vi "KPRO_2016_DPT2.vi"() -> ()   [LabVIEW 2016]
uses:
  Kpro Globals.vi
  <vilib>/Utility/file.llb/Write To Spreadsheet File (DBL).vi
panel:
  in  "Record DTW":bool
  out "Depth to Water":dbl=-30.877198474121087 format="%.2f"
  in  "In-Line Pressure Offset":dbl format="%.2f"
  in  "Zero In-Line Pressure\n(F = leave as is)":bool=TRUE
  in  "In-Line Pressure Slope":dbl=42.0 format="%.2f"
  out "In-Line Pressure":dbl=69.7228 format="%.2f"
  out "Drive Rate":dbl=16.666666666666664 format="%.2f"
  out "Real Time - Depth vs. Drive":cluster{dbl[], dbl[]}(graph)={[0.02036245163917736, 0.125, 0.16666666666666674, 0.16666666666666663, 0.16666666666666663, 0.16666666666666663], [-100.1, -100.2, -100.3, -100.4, -100.5, -100.6]}
  out "Current Depth (m)":sgl=-30.661383 format="%.2f"
  out "Zeroed \nPressure (m)":dbl=22.78027421497274 format="%.2f"
  out "Ik":dbl=0.003788962123473114 format="%.2f"
  in  "Hole_name_file":path=path "C:/e"
  in  "Output File KPRO Test":path=path "C:/e_KPRO.txt"
  in  "Output File Slug Test":path=path "C:/e_SLUG.txt"
  in  "Output File YSI Test":path=path "C:/e_YSI.txt"
  in  "Output File IK for GMS":path=path "C:/e_IKMGS.txt"
  in  "enable_IKMGS_file":bool
  in  "enable_slug_file":bool
  in  "enable_kpro_file":bool=TRUE
  out "Ik":dbl=0.003788962123473114 format="%.2f"
  out "Zeroed Pressure":dbl=74.74207969932556 format="%.2f"
  out "Current Depth":sgl=-100.6 format="%.2f"
  out "Flow":dbl=0.21081600494384767 format="%.2f"
  out "Real Time - Depth vs. lk":cluster{dbl[], dbl[]}(graph)={[0.003788962123473114, 0.0037174584307500765, 0.0037174584307500765, 0.0037174584307500765, 0.0037174584307500765, 0.003788962123473114], [-100.1, -100.2, -100.3, -100.4, -100.5, -100.6]}
  out "Hole_Name_Path":path=path "C:/e"
  in  "data_directory":string="C:\\KPRO_DATA\\SITE_NAME\\"
  out "Real Time - Depth vs. lk":cluster{dbl[], dbl[]}(graph)={[0.003788962123473114, 0.0037174584307500765, 0.0037174584307500765, 0.0037174584307500765, 0.0037174584307500765, 0.003788962123473114], [-100.1, -100.2, -100.3, -100.4, -100.5, -100.6]}
  in  "Reservoir Pressure":dbl=-0.004827000045779073 format="%.2f"
  in  "Simulate AD6B":bool
  in  "Atmospheric Pressure":dbl=32.22022530555725 format="%.2f"
  out "numrows":dbl format="%.2f"
  in  "Start\nYSI Capture":bool
  in  "Capture Head \nPressure":bool
  in  "Depth mode":bool caption="Use \nIncrement"
  out "Real Time - Depth vs. Drive":cluster{dbl[], dbl[]}(graph)={[0.02036245163917736, 0.125, 0.16666666666666674, 0.16666666666666663, 0.16666666666666663, 0.16666666666666663], [-100.1, -100.2, -100.3, -100.4, -100.5, -100.6]}
  out "Cumulative - Depth vs. Drive":cluster{dbl[], dbl[]}(graph)
  in  "Feet of Stainless":i32=40
  out "Slug Test\nIndicator":bool
  out "KPRO Test\nIndicator":bool
  in  "Increment\nButton":bool
  in  "Start\nST":bool
  in  "Zero\nPressure":bool
  out "Zeroed \nPressure":dbl=74.74207969932556 format="%.2f"
  in  "Finish Tests":bool
  out "Current Depth":sgl=-100.6 format="%.2f"
  in  "Start\nKPRO":bool
  out "Total Volume":dbl format="%.2f"
  in  "Clear \nTotal\nVolume":bool
  in  "Client ID - Not Used":string
  out "Flow":dbl=0.21081600494384767 format="%.2f"
  out "Cumulative - Depth vs. Ik":cluster{dbl[], dbl[]}(graph)
  # "Use new slope/offset"
  # "KPRO  DATALOGGER"
  # "STONE  ENVIRONMENTAL  2010"
  # "ON"
  # "OFF"
  # "String Pot"
  # "Revision History\n\nAdded metric depth and pressure - VLD - 12-20-07\nAdded Static Ik button and drive rate- VLD 1-28-10"
  # "Use Incr"
  # "ON"
  # "OFF"
  # "ON"
  # "OFF"
  # "ON"
  # "OFF"
  # "ON"
  # "OFF"
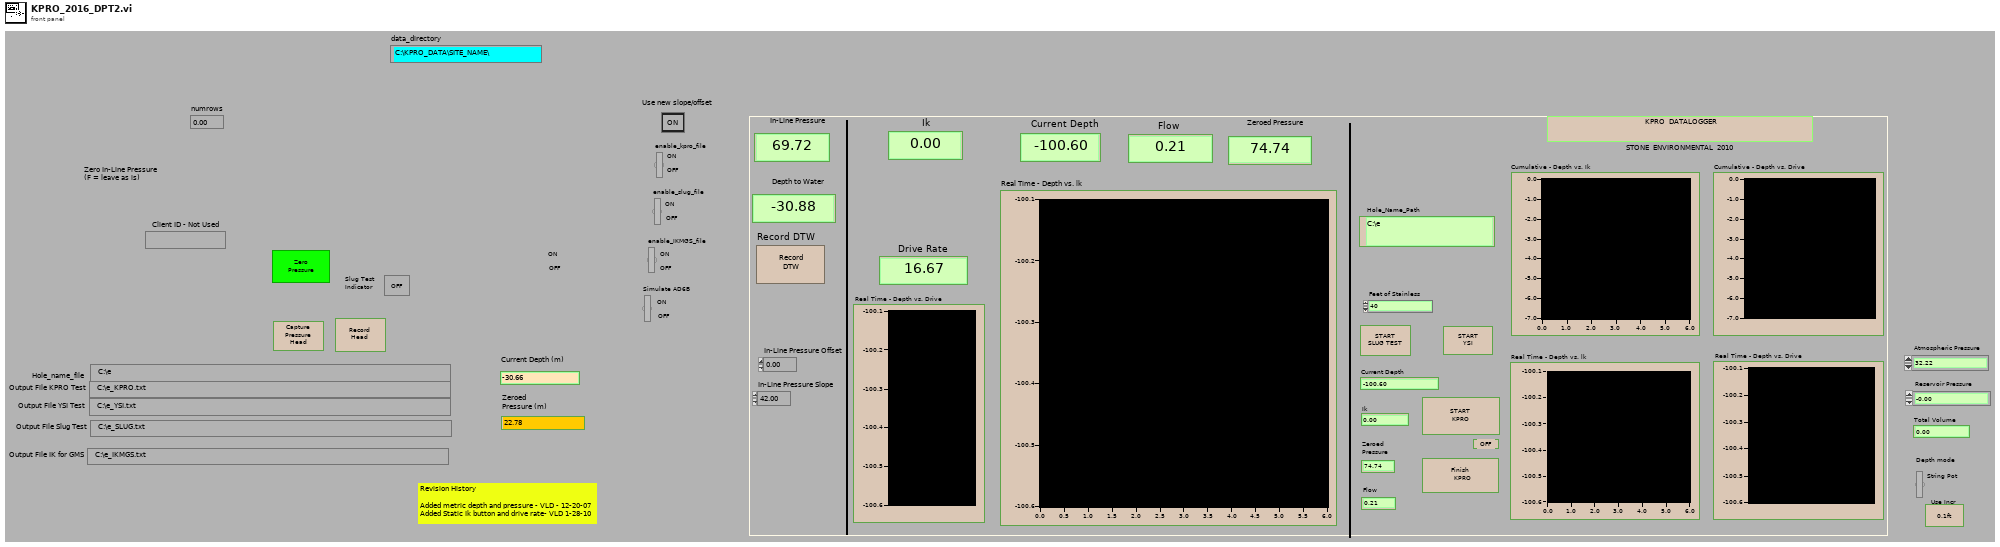
[diagram p1: front panel]
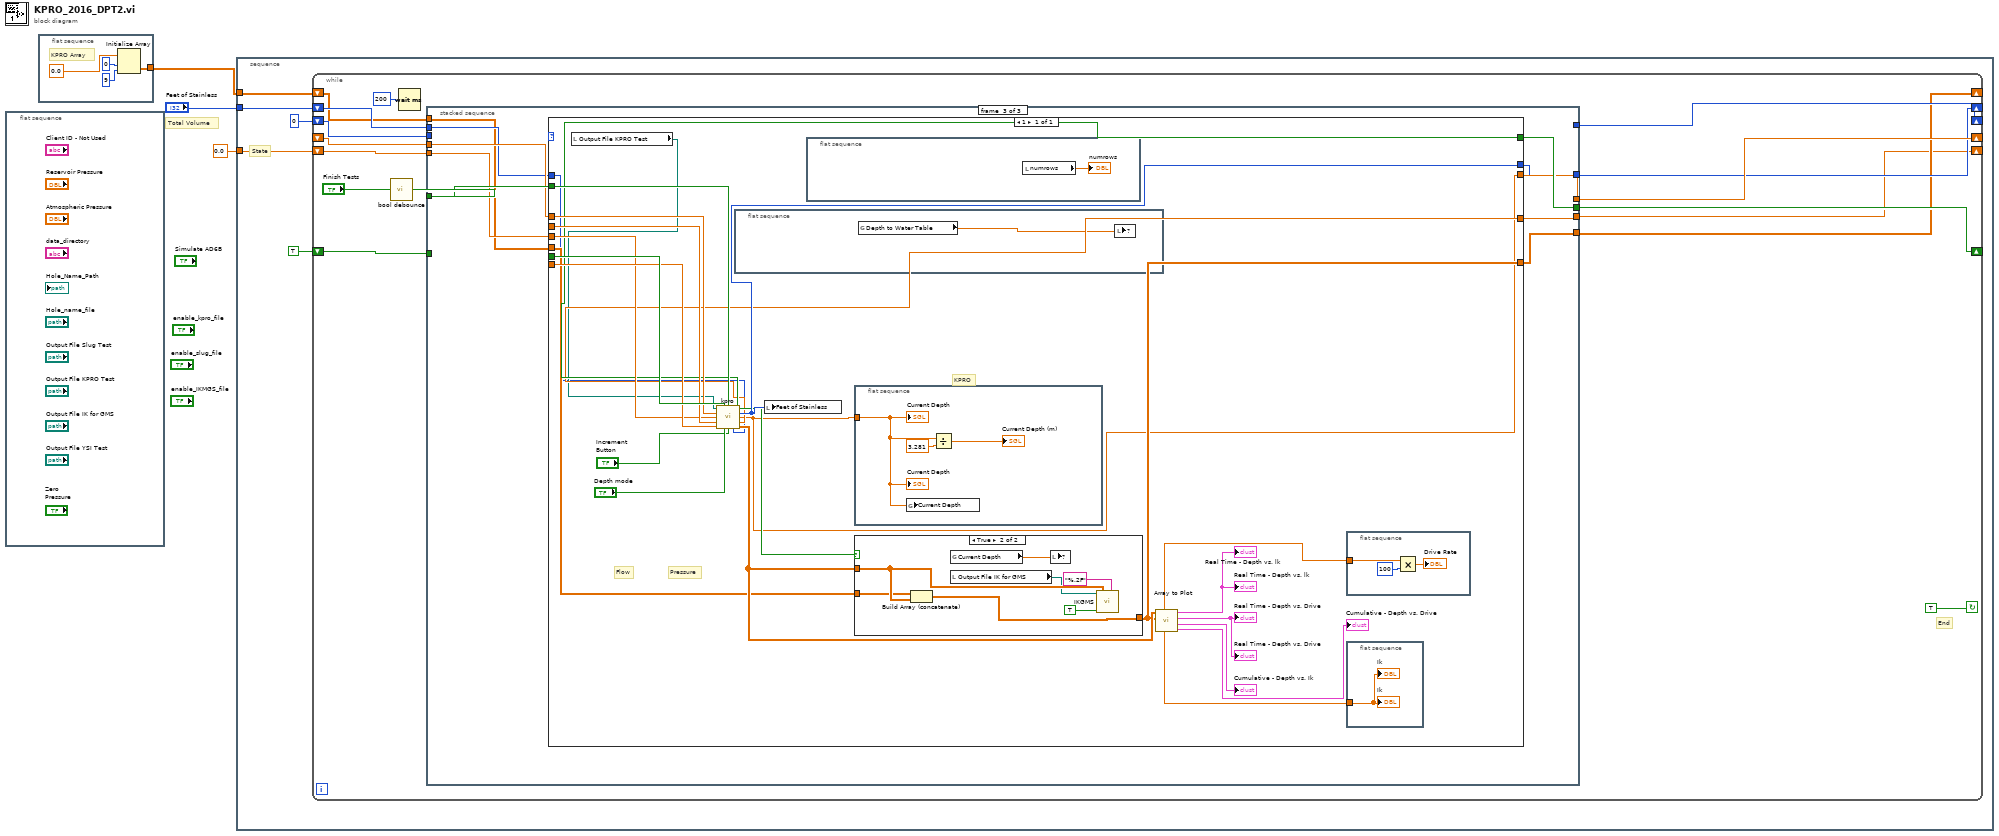
[diagram p0: block diagram]
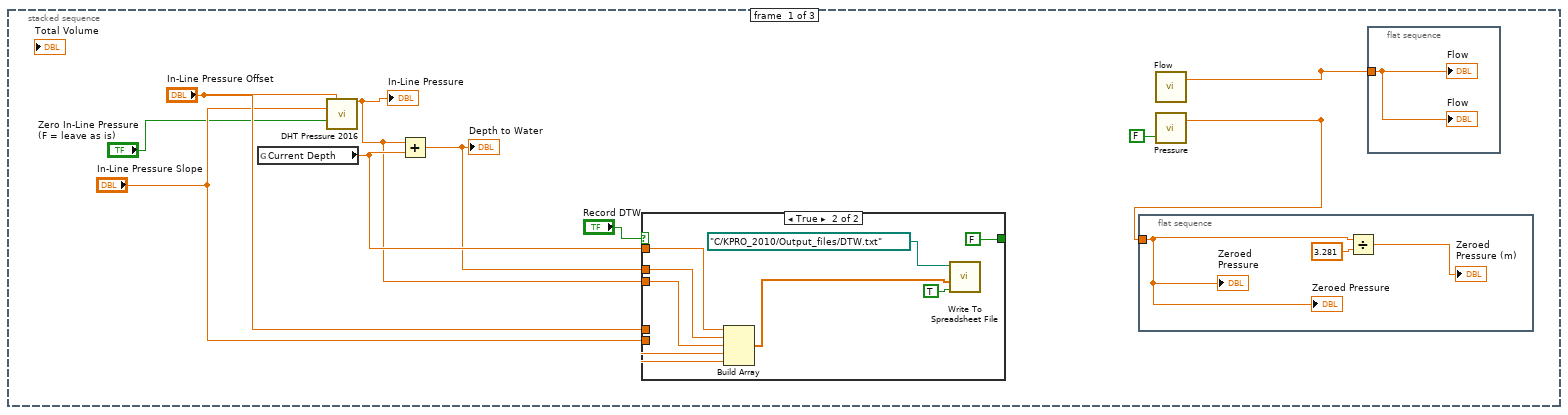
[diagram p2: hidden frame]
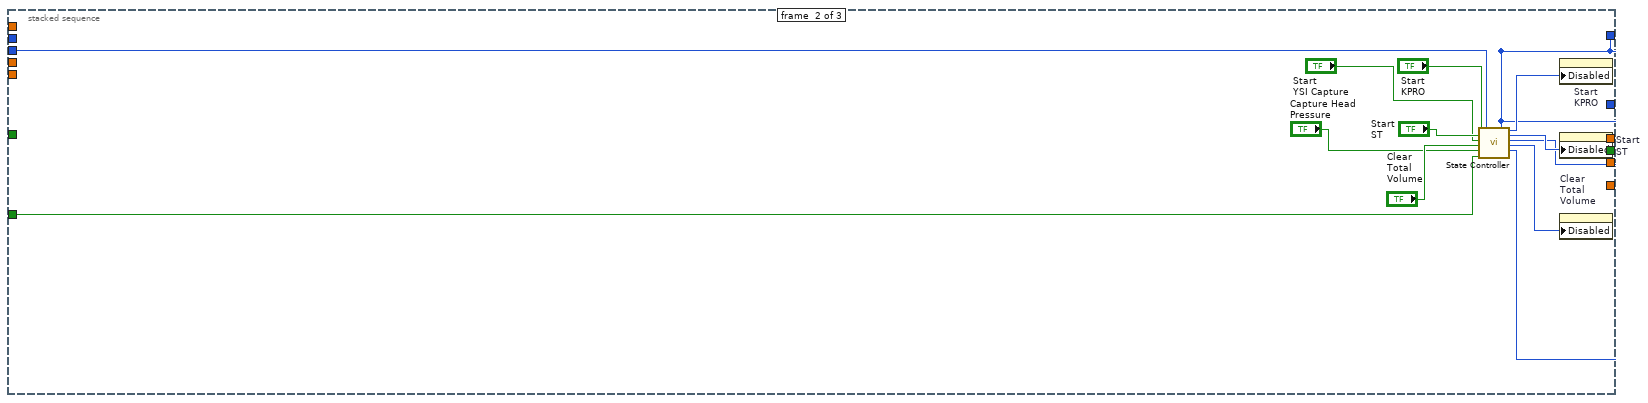
[diagram p4: hidden frame]
diagram:
  # "Total Volume"
  n1 = flat-sequence {
    frame #0 {
    }
  }
  n2 = flat-sequence {
    tunnel: [w4] -> w1
    frame #0 {
      # "KPRO Array"
      n3 = Initialize Array(0.0, 0, 9) -> (w4:dbl[][])
    }
  }
  n4 = stacked-sequence {
    tunnel: "Feet of Stainless" -> [w10]
    tunnel: 0.0 -> [w9]
    tunnel: w1 -> [w8]
    frame #0 {
      # "End"
      # "State"
      n5 = while {
        shift-left: w8 -> [w19]
        shift-right: [w18] -> _
        shift-left: w10 -> [w21]
        shift-right: [w20] -> _
        shift-left: _ -> [w24]
        shift-right: [w23] -> _
        shift-left: w9 -> [w22]
        shift-right: [w17] -> _
        shift-left: TRUE -> [w27]
        shift-right: [w26] -> _
        shift-left: 0 -> [w28]
        shift-right: [w25] -> _
        stop <- TRUE continue-if-true
        n6 = call "bool debounce.vi"("Input Boolean"="Finish Tests") -> ("Output Boolean"=w15:bool)
        n7 = Wait (ms)(milliseconds to wait=u32 200) -> ()  [unwired: 1 out]
        n8 = stacked-sequence {
          seq-local: [_ w53 _] -> [_ _ w85]
          seq-local: [_ w64 _] -> [_ _ w84]
          seq-local: [w37 _ _] -> [_ _ w82]
          seq-local: [w38 _ _] -> [_ _ w81]
          tunnel: w28 -> [_ w66 _]
          tunnel: w27 -> [_ w65 _]
          tunnel: [_ _ w86] -> w26
          tunnel: [_ w53 _] -> w25
          tunnel: w15 -> [_ _ w83]
          tunnel: w24 -> [_ _ w80]
          tunnel: [_ _ w79] -> w23
          tunnel: w22 -> [_ _ w78]
          tunnel: [_ _ w77] -> w17
          tunnel: w21 -> [_ _ w76]
          tunnel: [_ _ w75] -> w20
          tunnel: w19 -> [_ _ w74]
          tunnel: [_ _ w73] -> w18
          frame #0 {
            n9 = global read "Kpro Globals.vi" "Current Depth"() -> (w36:sgl)
            n10 = call "DHT Pressure 2016.vi"("DHT Pressure Offset"="In-Line Pressure Offset", "DHT Pressure \nSlope"="In-Line Pressure Slope", "Zero Pressure\n(F = leave as is)"="Zero In-Line Pressure\n(F = leave as is)") -> ("DHT Pressure"=w30:dbl)  [unwired: 10 in, 2 out]
            "In-Line Pressure" <- w30
            n11 = Add(x=w30, y=w36) -> (x+y=w34:dbl)
            "Depth to Water" <- w34
            n12 = case shown="True" "Record DTW" {
              selector: "Record DTW" -> [w43 _]
              tunnel: [w43 FALSE ("Boolean")] -> _
              tunnel: w34 -> [_ w47]
              tunnel: w36 -> [_ w48]
              tunnel: "In-Line Pressure Offset" -> [_ w45]
              tunnel: w30 -> [_ w46]
              tunnel: "In-Line Pressure Slope" -> [_ w44]
              frame False {
              }
              frame True {
                n13 = Build Array(w48, w47, w46, w45, w44) -> (w52:dbl[])
                n14 = call-poly <vilib>:"Write To Spreadsheet File.vi"("append to file? (new file:F)"=TRUE, "1D data"=w52, "file path (dialog if empty)"=path "C:/KPRO_2010/Output_files/DTW.txt") -> ()  [unwired: 5 in, 1 out]
              }
            }
            n15 = flat-sequence {
              tunnel: w37 -> [w42]
              frame #0 {
                n16 = Divide(x=w42, y=3.281) -> (x/y=→"Zeroed \nPressure (m)":dbl)
                "Zeroed \nPressure" <- w42
                "Zeroed Pressure" <- w42
              }
            }
            n17 = call "Flow.vi"() -> ("Flow (ml/min)"=w38:dbl)  [unwired: 3 in]
            n18 = call "Pressure.vi"("Zero Pressure\n(F = leave as is)"=FALSE ("Zero Pressure\n(F = leave as is)")) -> ("Pressure"=w37:dbl)  [unwired: 2 in]
            n19 = flat-sequence {
              tunnel: w38 -> [w39]
              frame #0 {
                "Flow" <- w39
                "Flow" <- w39
              }
            }
          }
          frame #1 {
            n20 = call "State Controller.vi"("Start KPRO"="Start\nKPRO", "Start Slug Test"="Start\nST", "Start YSI Capture"="Start\nYSI Capture", "Clear Volume"="Clear \nTotal\nVolume", "Capture Head Pressure"="Capture Head \nPressure", "Done"=w65, "Previous \nState"=w66) -> ("Next State"=w53:i32, "State Changed"=w64:bool, "Start KPRO Enabler"=w58:u8, "Start Slug Test Enabler"=w57:u8, "Start YSI Capture Enabler"=w56:u8, "Clear Volume Enabler"=w55:u8, "Capture Head Pressure Enabler"=w54:u8)  [unwired: 4 in, 2 out]
            n21 = property on="Start\nKPRO" class="Bool"("Disabled"=w58) -> ()  [unwired: 2 in, 2 out]
            n22 = property on="Start\nST" class="Bool"("Disabled"=w57) -> ()  [unwired: 2 in, 2 out]
            n23 = property on="Clear \nTotal\nVolume" class="Bool"("Disabled"=w55) -> ()  [unwired: 2 in, 2 out]
            n24 = flat-sequence {
              tunnel: w53 -> [w67]
              frame #0 {
                n25 = Equal?(x=w67, y=2) -> (x = y?=→"Slug Test\nIndicator":bool)
              }
            }
            n26 = flat-sequence {
              tunnel: w53 -> [w70]
              frame #0 {
                n27 = Equal?(x=w70, y=1) -> (x = y?=→"KPRO Test\nIndicator":bool)
              }
            }
            n28 = property on="Start\nYSI Capture" class="Bool"("Disabled"=w56) -> ()  [unwired: 2 in, 2 out]
            n29 = property on="Capture Head \nPressure" class="Bool"("Disabled"=w54) -> ()  [unwired: 2 in, 2 out]
          }
          frame #2 {
            # "Flow"
            # "Pressure"
            n30 = case shown="1" w85 {
              tunnel: [w100] -> w86
              tunnel: w84 -> [w109]
              tunnel: w83 -> [w108]
              tunnel: w82 -> [w107]
              tunnel: w81 -> [w106]
              tunnel: w80 -> [w105]
              tunnel: [w90] -> w79
              tunnel: w78 -> [w104]
              tunnel: [w95] -> w77
              tunnel: w76 -> [w87]
              tunnel: [w101] -> w75
              tunnel: w74 -> [w94]
              tunnel: [w98] -> w73
              frame 1 {
                # "KPRO"
                n31 = local read "Output File KPRO Test"() -> (w93:path)
                n32 = call "kpro.vi"("Output KPRO"=w93, "Initialize"=w109, "Finished In"=w108, "Absolute Depth In"=w105, "Total Volume in"=w104, "Zeroed Pressure"=w107, "Flow"=w106, "Read String Pot"="Depth mode", "Increment"="Increment\nButton", "SS In"=w87) -> ("Finished Out"=w100:bool, "SS Out"=w101:i32, "Current Depth Out"=w90:sgl, "Total Volume Out"=w95:dbl, "Output Array"=w99:dbl[][])  [unwired: 1 in]
                n33 = flat-sequence {
                  frame #0 {
                    n34 = global read "Kpro Globals.vi" "Depth to Water Table"() -> (w111:dbl)
                    n35 = local write item#-1(w111) -> ()
                  }
                }
                n36 = local write "Feet of Stainless"(w101) -> ()
                n37 = flat-sequence {
                  frame #0 {
                    n38 = local read "numrows"() -> (→"numrows":dbl)
                  }
                }
                n39 = flat-sequence {
                  tunnel: w90 -> [w114]
                  frame #0 {
                    n40 = global write "Kpro Globals.vi" "Current Depth"(w114) -> ()
                    n41 = Divide(x=w114, y=3.281) -> (x/y=→"Current Depth (m)":dbl)
                    "Current Depth" <- w114
                    "Current Depth" <- w114
                  }
                }
                n42 = case shown="True" w100 {
                  tunnel: [w119 w126] -> w98
                  tunnel: w99 -> [_ w125]
                  tunnel: w94 -> [w119 w121]
                  frame False {
                  }
                  frame True {
                    n43 = Build Array (concatenate)(w121, w125) -> (w126:dbl[][])
                    n44 = global read "Kpro Globals.vi" "Current Depth"() -> (w120:sgl)
                    n45 = local read "Output File IK for GMS"() -> (w123:path)
                    n46 = local write item#-1(w120) -> ()
                    n47 = call "IKGMS.vi"("format (%.3f)"="%.2F", "append to file? (new file:F)"=TRUE, "2D data"=w125, "file path (dialog if empty)"=w123) -> ()  [unwired: 4 in, 1 out]
                  }
                }
                n48 = call "Array to Plot.vi"("Input Cumulative Array"=w98, "Input Real Time Array"=w99) -> ("Cumulative - Depth vs.Drive Rate"=→"Cumulative - Depth vs. Drive":cluster{dbl[], dbl[]}, "Cumulative - Depth vs. Ik"=→"Cumulative - Depth vs. Ik":cluster{dbl[], dbl[]}, "Real Time - Depth vs. Drive Rate"=→"Real Time - Depth vs. Drive" →"Real Time - Depth vs. Drive":cluster{dbl[], dbl[]}, "Real Time - Depth vs. Ik"=→"Real Time - Depth vs. lk" →"Real Time - Depth vs. lk":cluster{dbl[], dbl[]}, "Current Ik"=w89:dbl, "Depth Rate"=w88:dbl)  [unwired: 2 in]
                n49 = flat-sequence {
                  tunnel: w88 -> [w117]
                  frame #0 {
                    n50 = Multiply(x=w117, y=100) -> (x*y=→"Drive Rate":dbl)
                  }
                }
                n51 = flat-sequence {
                  tunnel: w89 -> [w110]
                  frame #0 {
                    "Ik" <- w110
                    "Ik" <- w110
                  }
                }
              }
            }
          }
        }
      }
    }
  }
